vi "Slip cycle logic.vi"(0 "Trigger pulse (pos. edge)":bool, 5 "Wait Count":u16, 9 "AOD fill in":u16, 13 "Num_pixels_slip_cycle":u32, 14 "add_cycle":bool) -> (4 "AOD fill out":u16)   [LabVIEW 2020]
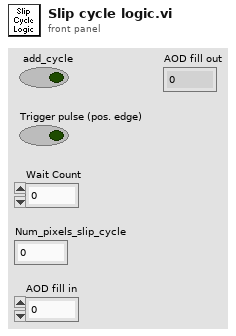
[diagram p1: front panel]
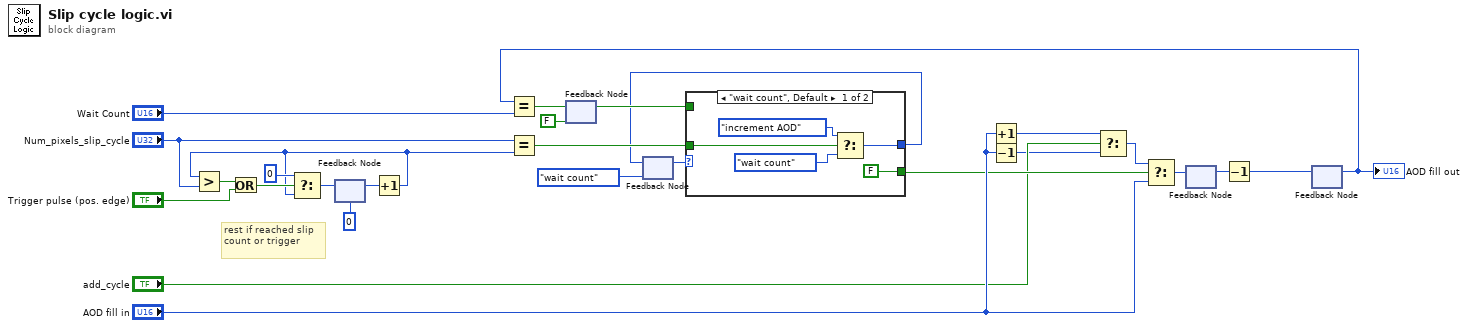
[diagram p0: block diagram]
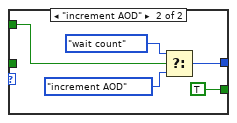
[diagram p2: hidden frame]
diagram:
  # "rest if reached slip count or trigger"
  n1 = feedback #1(u32 0) -> (w25:u32)
  n2 = Increment(x=w25) -> (x+1=w1:u32)
  n3 = Greater?(x=w1, y="Num_pixels_slip_cycle") -> (0:w4:bool)
  n4 = Or(x=w4, y="Trigger pulse (pos. edge)") -> (x .or. y?=w6:bool)
  n5 = Select(t=u32 0, s=w6, f=w1) -> (s? t:f=w27:u32)
  n6 = feedback-in #1(w27) -> ()
  n7 = Equal?(x="Num_pixels_slip_cycle", y=w1) -> (x = y?=w16:bool)
  n8 = feedback #2(FALSE) -> (w21:bool)
  n9 = feedback #3(enum16{"wait count", "increment AOD", ""}."wait count") -> (w13:enum16{"wait count", "increment AOD", ""})
  n10 = case shown="\"wait count\", Default" w13 {
    tunnel: [FALSE TRUE] -> w23
    tunnel: w16 -> [w32 _]
    tunnel: [w29 w33] -> w15
    tunnel: w21 -> [_ w34]
    frame "wait count", Default {
      n11 = Select(t=enum16{"wait count", "increment AOD", ""}."increment AOD", s=w32, f=enum16{"wait count", "increment AOD", ""}."wait count") -> (s? t:f=w29:enum16{"wait count", "increment AOD", ""})
    }
    frame "increment AOD" {
      n12 = Select(t=enum16{"wait count", "increment AOD", ""}."wait count", s=w34, f=enum16{"wait count", "increment AOD", ""}."increment AOD") -> (s? t:f=w33:enum16{"wait count", "increment AOD", ""})
    }
  }
  n13 = feedback-in #3(w15) -> ()
  n14 = Increment(x="AOD fill in") -> (x+1=w8:u16)
  n15 = Decrement(x="AOD fill in") -> (x-1=w9:u16)
  n16 = Select(t=w8, s="add_cycle", f=w9) -> (s? t:f=w12:u16)
  n17 = Select(t=w12, s=w23, f="AOD fill in") -> (s? t:f=w22:u16)
  n18 = feedback #4() -> (w11:u16)  [unwired: 1 in]
  n19 = feedback-in #4(w22) -> ()
  n20 = Decrement(x=w11) -> (x-1=w18:u16)
  n21 = feedback #5() -> (w5:u16)  [unwired: 1 in]
  "AOD fill out" <- w5
  n22 = Equal?(x=w5, y="Wait Count") -> (x = y?=w17:bool)
  n23 = feedback-in #2(w17) -> ()
  n24 = feedback-in #5(w18) -> ()
